vi "Validate Build Spec.vi"(7 "Build object type":T1, 8 "error in (no error)":errorcluster, 9 "Build spec name":string, 11 "TargetItem in":refnum<vi>) -> (0 "error out":errorcluster, 1 "Build spec name dup":string, 3 "TargetItem out":refnum<vi>, 4 "Valid":bool)   [LabVIEW 2012]
uses:
  <vilib>/AppBuilder/AB_API/common/AB_API Build Object Type.ctl
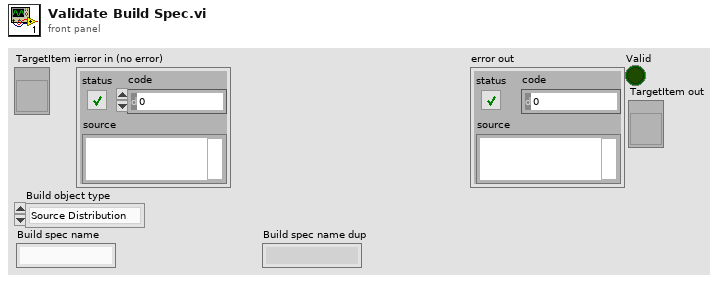
[diagram p1: front panel]
types:
  T1 = typedef "AB_API Build Object Type.ctl" = enum16{"Source Distribution", "DLL", "EXE", "Installer", "Zip File", "RESTful WS", "RTEXE", "Packed Library", "C Generation "}
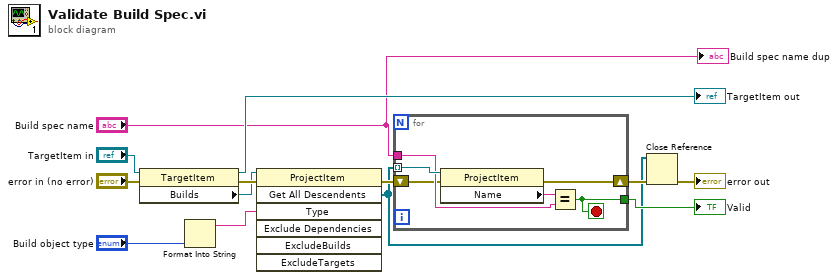
[diagram p0: block diagram]
diagram:
  n1 = property class="TargetItem"(reference="TargetItem in", error in="error in (no error)") -> (reference out=→"TargetItem out":refnum<vi>, error out=w9:errorcluster, "Builds"=w8:refnum<vi>)
  n2 = Format Into String("Build object type") -> (resulting string=w10:string)  [unwired: 3 in, 1 out]
  n3 = invoke class="ProjectItem" method="Get All Descendents"(reference=w8, error in=w9, "Type"=w10) -> (error out=w7:errorcluster, "All Descendents"=w2:refnum<vi>[])  [unwired: 4 in, 5 out]
  n4 = for {
    tunnel: w2 -> [w19] mode=indexing
    tunnel: "Build spec name" -> [w17]
    tunnel: [w16] -> w5
    shift-right: [w14] -> w6
    shift-left: w7 -> [w15]
    stop <- w16 stop-if-true
    n5 = property class="ProjectItem"(reference=w19, error in=w15) -> (error out=w14:errorcluster, "Name"=w18:string)  [unwired: 1 out]
    n6 = Equal?(x=w18, y=w17) -> (x = y?=w16:bool)
  }
  "Valid" <- w5
  n7 = Close Reference(reference=w2, error in (no error)=w6) -> (error out=→"error out":errorcluster)
  "Build spec name dup" <- "Build spec name"
